vi "classify error.vi"(8 "error to classify":errorcluster, 11 "fixed channel runtime in":refnum<class "control module runtime.lvclass">) -> (0 "classified error":errorcluster, 2 "error classification":T1, 3 "fixed channel runtime out":refnum<class "control module runtime.lvclass">)   [LabVIEW 2013, in "control module runtime.lvclass"]
doc: "Allows a module to classify an error generated at any point during execution. This <b>error classification</b> can then be used by calling code to determine if execution can continue. In addition, this function can be used to allow a component to clear an error, convert an error to a warning, or attempt to recover from an error. Recovery may be attempted only if <b>attempt recovery?</b> is true."
uses:
  control module runtime.lvclass
  <vilib>/NI/Tag Bus Module Framework/runtime/error classification.ctl
  control module runtime.lvclass/control module runtime.ctl
  <vilib>/NI/Tag Bus Module Framework/runtime/TBM module execution interface.lvclass
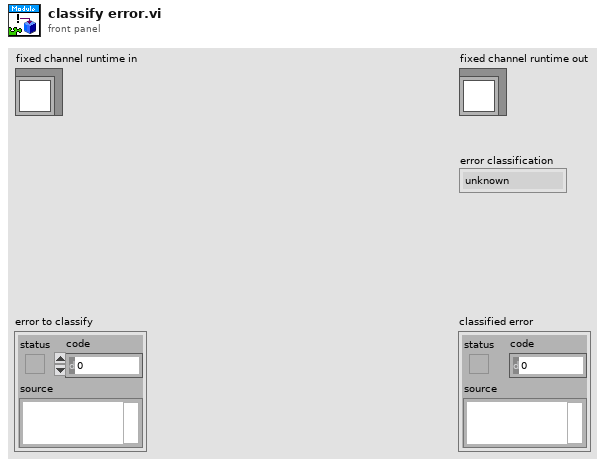
[diagram p1: front panel]
types:
  T1 = typedef "TBM module execution interface.lvclass/error classification.ctl" = enum16{"unknown", "none", "trivial", "recoverable", "critical"}
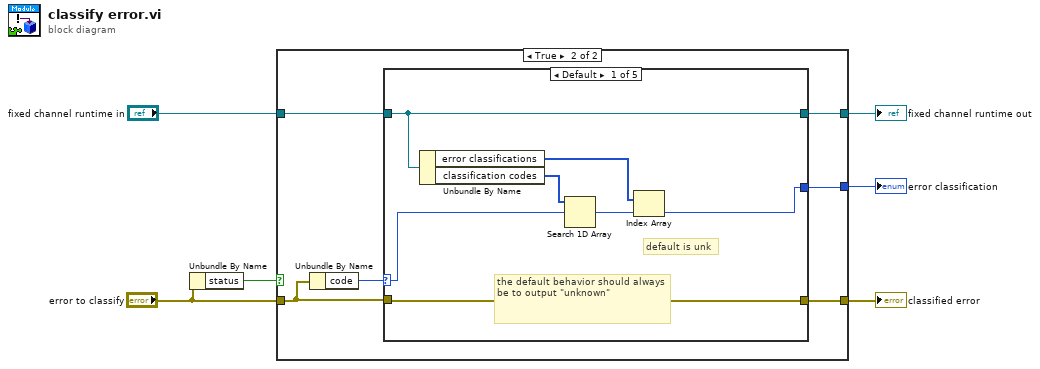
[diagram p0: block diagram]
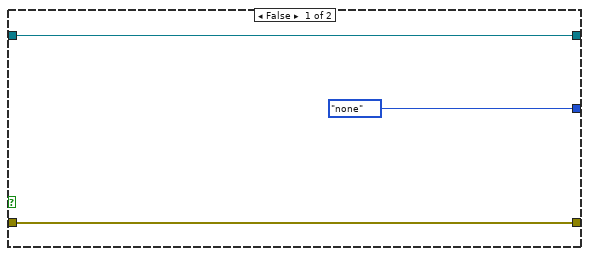
[diagram p2: hidden frame]
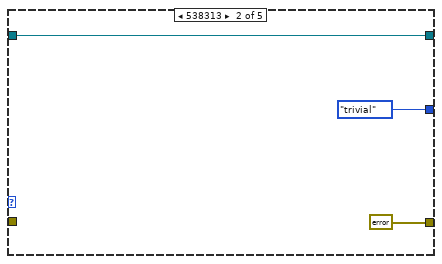
[diagram p3: hidden frame]
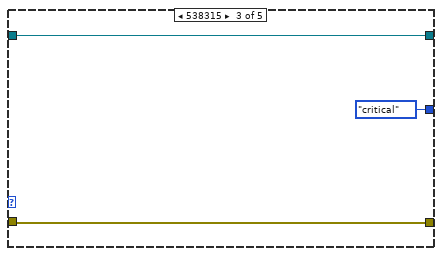
[diagram p4: hidden frame]
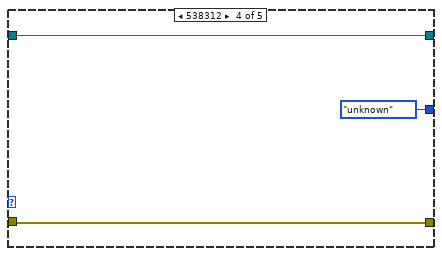
[diagram p5: hidden frame]
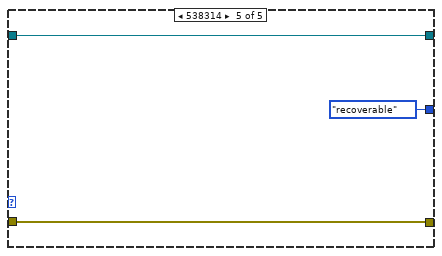
[diagram p6: hidden frame]
diagram:
  n1 = Unbundle By Name("error to classify") -> ("status"=w2:bool)
  n2 = case shown="True" w2 {
    tunnel: [w9 w11] -> w6
    tunnel: "fixed channel runtime in" -> [w9 w12]
    tunnel: [w7 w14] -> w4
    tunnel: [error_classification."none" ("error classification") w13] -> w3
    tunnel: "error to classify" -> [w7 w10]
    frame False {
    }
    frame True {
      n3 = Unbundle By Name(w10) -> ("code"=w15:i32)
      n4 = case shown="Default" w15 {
        selector: w15 -> [w19 _ _ _ _]
        tunnel: w10 -> [w22 _ w26 w29 w34]
        tunnel: [w22 errorcluster {"status"=FALSE, "code"=0, "source"=""} ("error constant") w26 w29 w34] -> w14
        tunnel: [w16 error_classification."trivial" ("error classification") error_classification."critical" ("error classification") error_classification."unknown" ("error classification") error_classification."recoverable" ("error classification")] -> w13
        tunnel: w12 -> [w21 w23 w28 w31 w32]
        tunnel: [w21 w23 w28 w31 w32] -> w11
        frame Default {
          # "the default behavior should always be to output \"unknown\""
          # "default is unk"
          n5 = Unbundle By Name(w21) -> ("error classifications"=w18:T1[], "classification codes"=w20:i32[])
          n6 = Search 1D Array(1D array=w20, element=w19) -> (index of element=w17:i32)  [unwired: 1 in]
          n7 = Index Array(array=w18, index=w17) -> (element=w16:T1)
        }
        frame 538313 {
        }
        frame 538315 {
        }
        frame 538312 {
        }
        frame 538314 {
        }
      }
    }
  }
  "fixed channel runtime out" <- w6
  "error classification" <- w3
  "classified error" <- w4
